vi "OnlinePic.vi"(6 "action":T2(ring), 7 "RGB/False":bool, 8 "Threshold (max)":cluster{"max":u32, "min":u32}, 9 "plane":u32, 10 "router channel":u8, 11 "Array":u32[][][][](array[numeric])) -> (0 "Title":string, 1 "Image Out (duplicate)":T1, 2 "Sum of Photons":u32[][][][](array[numeric]), 3 "RGB/False out":bool, 4 "Threshold (max) OUT":cluster{"max":u32, "min":u32})   [LabVIEW 2009]
uses:
  <vilib>/vision/Image Controls.llb/IMAQ Image.ctl
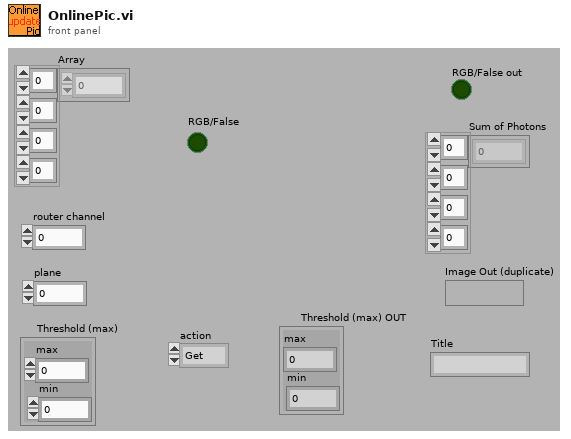
[diagram p1: front panel]
types:
  T1 = typedef "IMAQ Image.ctl" = refnum<image>
  T2 = enum16{"Get", "Set", "Change", "ini", "clear", "draw", "draw false"}
  T3 = enum16{"Get", "Set", "Change", "ini", "clear", "draw"}
  T4 = enum32{"No Selection", "Point", "Line", "Rectangle", "Oval", "Polygon", "Free", "Unused1", "Zoom", "Unused2", "Broken Line", "Free Hand Line"}[]
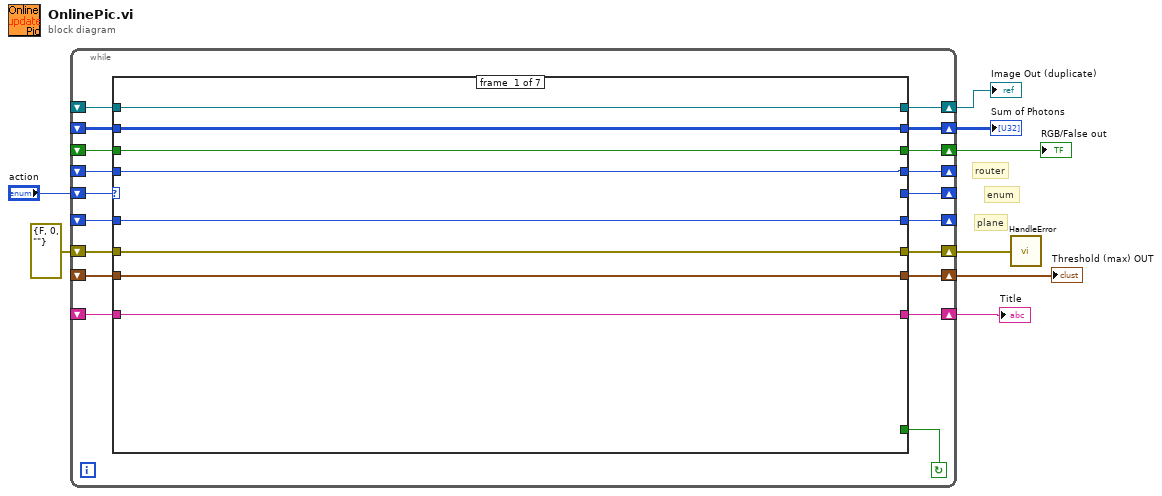
[diagram p0: block diagram]
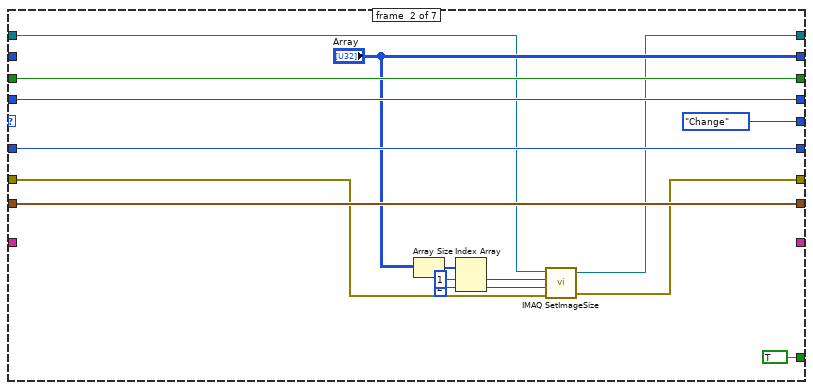
[diagram p2: hidden frame]
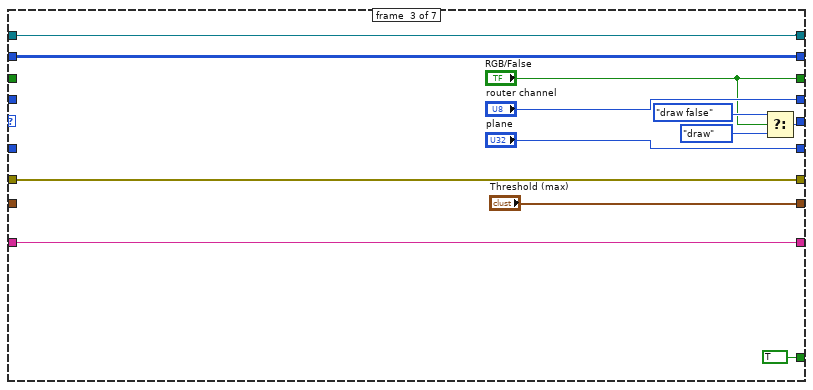
[diagram p3: hidden frame]
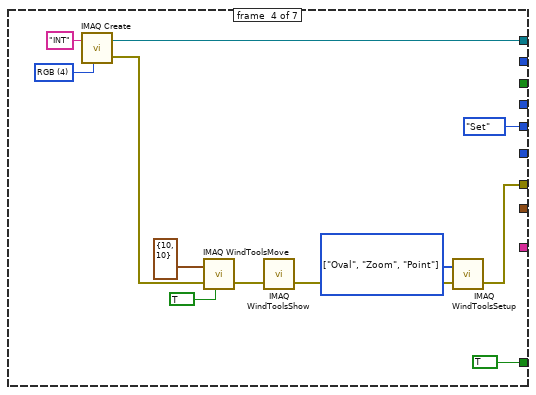
[diagram p4: hidden frame]
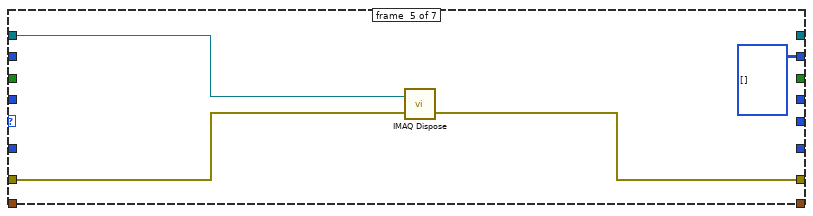
[diagram p5: hidden frame]
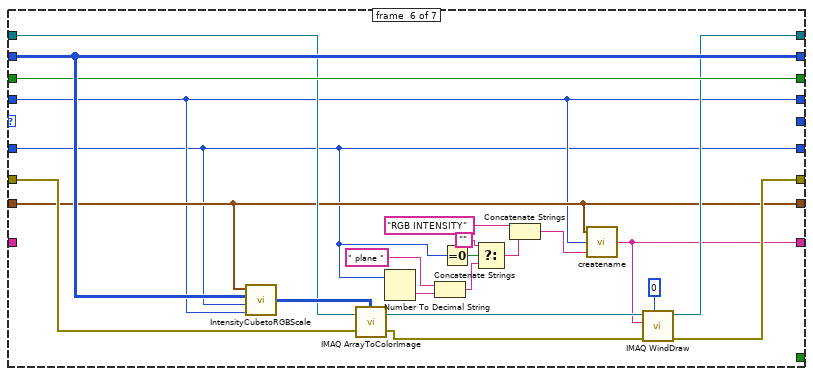
[diagram p6: hidden frame]
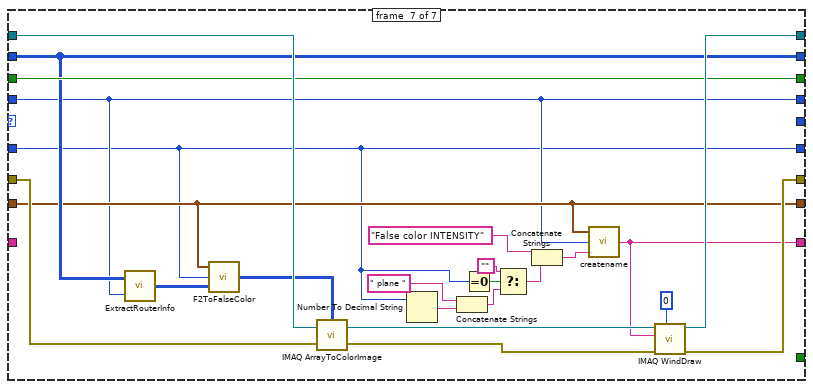
[diagram p7: hidden frame]
diagram:
  # "plane"
  # "enum"
  # "router"
  n1 = while {
    shift-right: [w18] -> w3
    shift-left: _ -> [w14]
    shift-right: [w24] -> w7
    shift-left: _ -> [w22]
    shift-right: [w26] -> w6
    shift-left: _ -> [w23]
    shift-right: [w17] -> _
    shift-left: _ -> [w13]
    shift-right: [w21] -> _
    shift-left: "action" -> [w27]
    shift-right: [w25] -> w1
    shift-left: errorcluster {"status"=FALSE, "code"=0, "source"=""} ("error out") -> [w19]
    shift-right: [w16] -> _
    shift-left: _ -> [w12]
    shift-right: [w15] -> w2
    shift-left: _ -> [w11]
    shift-right: [w9] -> w4
    shift-left: _ -> [w10]
    stop <- w20 continue-if-true
    n2 = case shown="\"draw\"" w27 {
      tunnel: [w35 w42 w59 w74 _ w94 w121] -> w26
      tunnel: [w30 w41 w56 w67 w77 w93 w119] -> w25
      tunnel: [w34 "Array" w63 _ u32[][][][] [] ("Array") w101 w114] -> w24
      tunnel: w23 -> [w35 w43 w59 _ w79 w95 w123]
      tunnel: w22 -> [w34 _ w63 _ _ w101 w114]
      tunnel: [_ T2."Change" ("Enum") w53 T3."Set" ("Enum") _ _ _] -> w21
      tunnel: [_ TRUE TRUE TRUE _ _ _] -> w20
      tunnel: w19 -> [w30 w40 w56 _ w78 w92 w118]
      tunnel: [w33 w47 "RGB/False" _ _ w100 w117] -> w18
      tunnel: [w32 w50 "router channel" _ _ w90 w112] -> w17
      tunnel: [w31 w49 "plane" _ _ w80 w103] -> w16
      tunnel: [w29 w48 "Threshold (max)" _ _ w91 w113] -> w15
      tunnel: w14 -> [w33 w47 _ _ _ w100 w117]
      tunnel: w13 -> [w32 w50 _ _ _ w90 w112]
      tunnel: w12 -> [w31 w49 _ _ _ w80 w103]
      tunnel: w11 -> [w29 w48 _ _ _ w91 w113]
      tunnel: w10 -> [w28 _ w57 _ _ _ _]
      tunnel: [w28 _ w57 _ _ w89 w111] -> w9
      frame #0 {
      }
      frame #1 {
        n3 = Array Size(array="Array") -> (size(s)=w44:i32[])
        n4 = Index Array(array=w44, index #1=1 ("index"), index #2=2 ("index")) -> (element #1=w39:i32, element #2=w38:i32)
        n5 = call "IMAQ SetImageSize"("error in (no error)"=w40, "Y Resolution"=w38, "X Resolution"=w39, "Image"=w43) -> ("error out"=w41:errorcluster, "Image Out"=w42:T1)  [unwired: 1 in]
      }
      frame #2 {
        n6 = Select(t=T2."draw false" ("Enum"), s="RGB/False", f=T2."draw" ("Enum")) -> (s? t:f=w53:T2)
      }
      frame #3 {
        w71 = T4 [enum."Oval", enum."Zoom", enum."Point"] items=["No Selection", "Point", "Line", "Rectangle", "Oval", "Polygon", "Free", "Unused1", "Zoom", "Unused2", "Broken Line", "Free Hand Line"] ("Tools")
        w75 = u32 4 items=["8 bits", "16 bits", "Float", "Complex", "RGB", "HSL"] ("Image Type")
        n7 = call "IMAQ Create"("Image Name"="INT", "Image Type"=w75) -> ("New Image"=w74:T1, "error out"=w66:errorcluster)  [unwired: 3 in]
        n8 = call "IMAQ WindToolsMove"("Coordinates"=cluster{"Y Position":i32, "X Position":i32} {"Y Position"=10, "X Position"=10}, "Get/Set Status? (Set)"=TRUE, "error in (no error)"=w66) -> ("error out"=w70:errorcluster)  [unwired: 2 in, 1 out]
        n9 = call "IMAQ WindToolsShow"("error in (no error)"=w70) -> ("error out"=w72:errorcluster)  [unwired: 4 in, 1 out]
        n10 = call "IMAQ WindToolsSetup"("Tools"=w71, "error in (no error)"=w72) -> ("error out"=w67:errorcluster)  [unwired: 4 in]
      }
      frame #4 {
        n11 = call "IMAQ Dispose"("Image"=w79, "error in (no error)"=w78) -> ("error out"=w77:errorcluster)  [unwired: 4 in]
      }
      frame #5 {
        n12 = call "IntensityCubetoRGBScale.vi"("Router"=w90, "Plane"=w80, "Trace"=w101, "threshold"=w91) -> ("RGB Scale"=w96:u32[][])
        n13 = call "IMAQ ArrayToColorImage"("Image Pixels (U32)"=w96, "Image"=w95, "error in (no error)"=w92) -> ("Image Out"=w98:T1, "error out"=w97:errorcluster)  [unwired: 2 in]
        n14 = Number To Decimal String(number=w80) -> (decimal integer string=w83:string)  [unwired: 1 in]
        n15 = Concatenate Strings(" plane " ("f"), w83) -> (w82:string)
        n16 = Equal To 0?(x=w80) -> (x = 0?=w86:bool)
        n17 = Select(t="", s=w86, f=w82) -> (s? t:f=w81:string)
        n18 = Concatenate Strings("RGB INTENSITY", w81) -> (w87:string)
        n19 = call "createname.vi"("Title"=w87, "router channel"=w90, "threshold"=w91) -> ("Title 2"=w89:string)
        n20 = call "IMAQ WindDraw"("Window Number (0...15)"=0, "error in (no error)"=w97, "Title"=w89, "Image"=w98) -> ("error out"=w93:errorcluster, "Image Out (duplicate)"=w94:T1)  [unwired: 6 in]
      }
      frame #6 {
        n21 = call "ExtractRouterInfo.vi"("router channel"=w112, "Array 2"=w114) -> ("Array"=w115:u32[][][][])
        n22 = call "F2ToFalseColor.vi"("Intensity"=w115, "Plane"=w103, "Threshold (max)"=w113) -> ("FalseColor"=w116:u32[][])
        n23 = call "IMAQ ArrayToColorImage"("Image Pixels (U32)"=w116, "Image"=w123, "error in (no error)"=w118) -> ("Image Out"=w122:T1, "error out"=w120:errorcluster)  [unwired: 2 in]
        n24 = Number To Decimal String(number=w103) -> (decimal integer string=w107:string)  [unwired: 1 in]
        n25 = Concatenate Strings(" plane " ("f"), w107) -> (w106:string)
        n26 = Equal To 0?(x=w103) -> (x = 0?=w110:bool)
        n27 = Select(t="", s=w110, f=w106) -> (s? t:f=w105:string)
        n28 = Concatenate Strings("False color INTENSITY", w105) -> (w102:string)
        n29 = call "createname.vi"("Title"=w102, "router channel"=w112, "threshold"=w113) -> ("Title 2"=w111:string)
        n30 = call "IMAQ WindDraw"("Window Number (0...15)"=0, "error in (no error)"=w120, "Title"=w111, "Image"=w122) -> ("error out"=w119:errorcluster, "Image Out (duplicate)"=w121:T1)  [unwired: 6 in]
      }
    }
  }
  "Sum of Photons" <- w7
  "Image Out (duplicate)" <- w6
  "Title" <- w4
  "RGB/False out" <- w3
  "Threshold (max) OUT" <- w2
  n31 = call "HandleError.vi"("error in (no error)"=w1) -> ()
